vi "alpha_sub.vi"(7 "alpha_pre":fxp<+/-,20,9>, 8 "ticks_m_pre":u32, 9 "ticks":u32, 10 "count_pre":i32, 11 "count":i32) -> (0 "ticks_m":u32, 3 "alpha":fxp<+/-,20,9>)   [LabVIEW 2014]
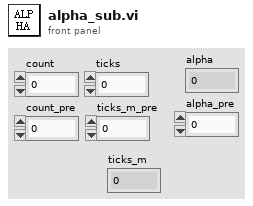
[diagram p1: front panel]
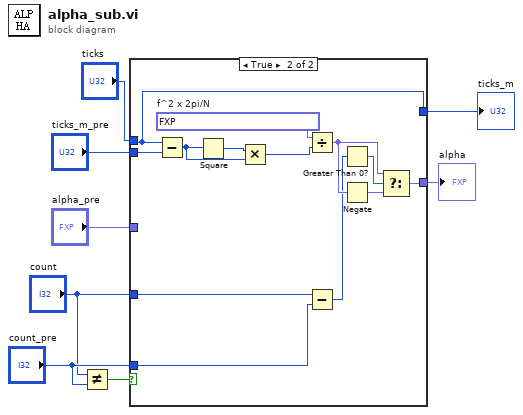
[diagram p0: block diagram]
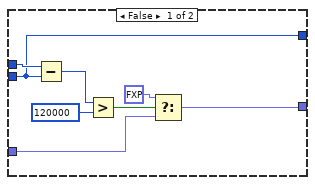
[diagram p2: hidden frame]
diagram:
  n1 = Not Equal?(x="count", y="count_pre") -> (x != y?=w8:bool)
  n2 = case shown="True" w8 {
    tunnel: "ticks" -> [w16 w21]
    tunnel: "count_pre" -> [_ w29]
    tunnel: [w15 w21] -> w1
    tunnel: "ticks_m_pre" -> [w15 w22]
    tunnel: [w11 w25] -> w6
    tunnel: "alpha_pre" -> [w12 _]
    tunnel: "count" -> [_ w23]
    frame False {
      n3 = Subtract(x=w16, y=w15) -> (x-y=w14:u32)
      n4 = Greater?(x=w14, y=u32 120000) -> (0:w13:bool)
      n5 = Select(t=fxp<+/-,20,9> 0.0, s=w13, f=w12) -> (s? t:f=w11:fxp<+/-,20,9>)
    }
    frame True {
      w20 = fxp<+,54,45> 2513274122871.83  # f^2 x 2pi/N
      n6 = Subtract(x=w21, y=w22) -> (x-y=w18:u32)
      n7 = Square(x=w18) -> (x^2=w19:u32)
      n8 = Multiply(x=w19, y=w18) -> (x*y=w17:u32)
      n9 = Divide(x=w20, y=w17) -> (x/y=w27:fxp<+/-,20,9>)
      n10 = Subtract(x=w23, y=w29) -> (x-y=w24:i32)
      n11 = Greater Than 0?(x=w24) -> (x > 0?=w26:bool)
      n12 = Negate(x=w27) -> (-x=w28:fxp<+/-,20,9>)
      n13 = Select(t=w27, s=w26, f=w28) -> (s? t:f=w25:fxp<+/-,20,9>)
    }
  }
  "alpha" <- w6
  "ticks_m" <- w1
